vi "RFID MFRC522 Example.vi"   [LabVIEW 2014]
doc: "This example shows how read/write data to RFID tag (MFRC522)"
uses:
  QwaveSys_Interface/QwaveSys_Interface.lvlib
  PWS_ESP8266/PWS_ESP8266.lvlib
panel:
  # "Overview: Demonstrates how to read communicate with contactless reader/writer RFID NXP MFRC522.\nRequirements: LabVIEW Full Development System,Arduino Compatible Compiler for LabVIEW,Programmable Wireless Stamp (PWS) Library.\nInstructions:\n1. Plug-in RFID MFRC522 module  to SPI port refer diagram below.\n2.  If this example has been loaded from the Arduino Compatible Compiler for LabVIEW, simply select Compile and Download.  Otherwise, open Tools>Arduino Compatible Compiler for LabVIEW in LabVIEW, then select File>Load VI, and select this VI and then Compile and Download.\n3. Open \"Serial Monitor\" by select \"Tools>Serial Monitor\" and select baud rate to 9600.\n4. Observe the logged data being print out on serial port monitor. \n\n#NOTE: \nThe MFRC522 is an integrated reader/writer integrated circuit for contactless communication at 13.56 MHz, by NXP technologies. refer : \"http://www.nxp.com/products/identification-and-security/nfc-and-reader-ics/nfc-frontend-solutions/standard-3v-mifare-reader-solution:MFRC522\""
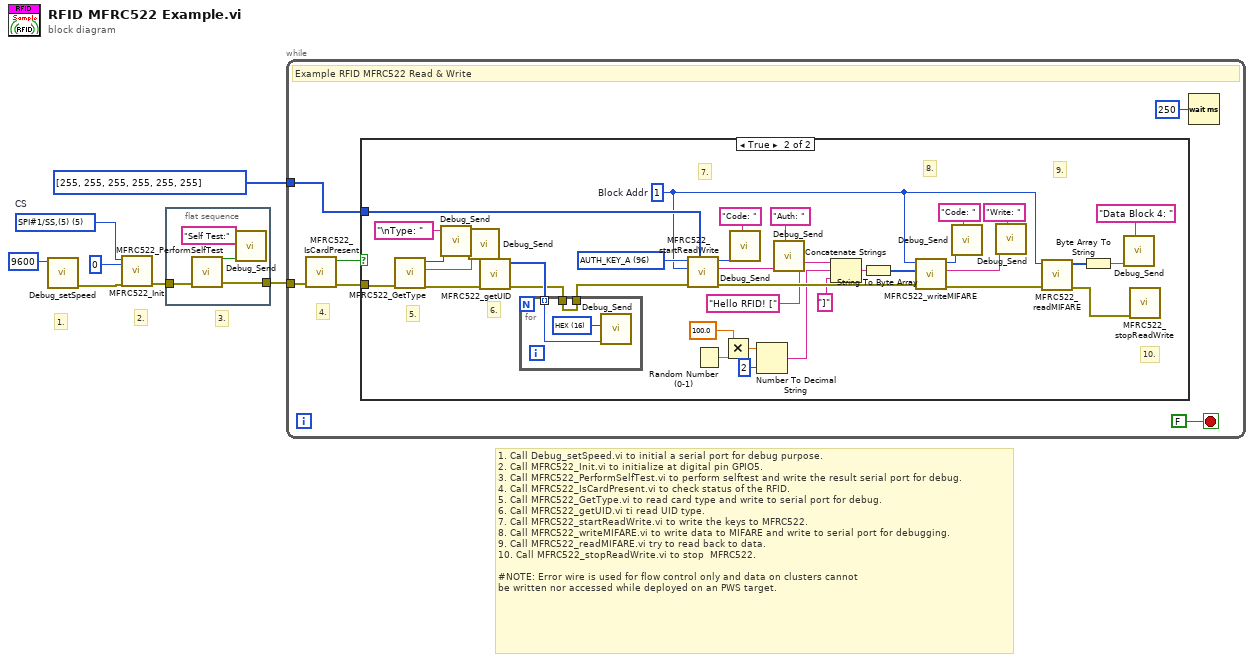
[diagram p0: block diagram]
diagram:
  w1 = u8 5 items=["SPI#1/SS,(5)"=5, "SPI#2/MOSI,(13)"=13, "SPI#3/MISO,(12)"=12, "SPI#4/SCLK,(14)"=14, "UART#1/CS,(15)"=15, "UART#2/TXD,(1)"=1, "UART#3/RXD,(3)"=3, "UART#4/LED,(16)"=16, "FPROM_Btn,(0)"=0, "SDCard_CS,(4)"=4, "I2C-SDA/TXD1,(2)"=2, "ADC0,(17)"=17]  # CS
  # "1. Call Debug_setSpeed.vi to initial a serial port for debug purpose.\n2. Call MFRC522_Init.vi to initialize at digital pin GPIO5.\n3. Call MFRC522_PerformSelfTest.vi to perform selftest and write the result serial port for debug.\n4. Call MFRC522_IsCardPresent.vi to check status of the RFID.\n5. Call MFRC522_GetType.vi to read card type and write to serial port for debug.\n6. Call MFRC522_getUID.vi ti read UID type.\n7. Call MFRC522_startReadWrite.vi to write the keys to MFRC522.\n8. Call MFRC522_writeMIFARE.vi to write data to MIFARE and write to serial port for debugging.\n9. Call MFRC522_readMIFARE.vi try to read back to data.\n10. Call MFRC522_stopReadWrite.vi to stop  MFRC522.\n\n#NOTE: Error wire is used for flow control only and data on clusters cannot\nbe written nor accessed while deployed on an PWS target."
  # "3."
  # "2."
  # "1."
  n1 = call "Debug_setSpeed.vi"("Speed"=u32 9600) -> ("error out"=w6:errorcluster)  [unwired: 10 in]
  n2 = call "MFRC522_Init.vi"("error in (no error)"=w6, "Reset"=u8 0, "Chip Select"=w1) -> ("error out"=w3:errorcluster)  [unwired: 8 in]
  n3 = flat-sequence {
    tunnel: w3 -> [w10]
    tunnel: [w9] -> w2
    frame #0 {
      n4 = call "MFRC522_PerformSelfTest.vi"("error in (no error)"=w10) -> ("error out"=w9:errorcluster, "status"=w8:bool)  [unwired: 9 in]
      n5 = call "Debug_Send.vi"("Name"="Self Test:", "DATA"=w8) -> ()  [unwired: 10 in]
    }
  }
  n6 = while {
    tunnel: w2 -> [w17]
    tunnel: u8[] [255, 255, 255, 255, 255, 255] ("Key (6 bytes)") -> [w12]
    stop <- FALSE stop-if-true
    # "4."
    # "Example RFID MFRC522 Read & Write"
    n7 = call "MFRC522_IsCardPresent.vi"("error in (no error)"=w17) -> ("error out"=w16:errorcluster, "status"=w13:bool)  [unwired: 9 in]
    n8 = case shown="True" w13 {
      tunnel: w16 -> [_ w36]
      tunnel: w12 -> [_ w49]
      frame False {
      }
      frame True {
        w18 = u8 1  # Block Addr
        w51 = u16 96 items=["AUTH_KEY_A"=96, "AUTH_KEY_B"=97] ("Key")
        # "10."
        # "9."
        # "8."
        # "7."
        # "6."
        # "5."
        n9 = call "MFRC522_GetType.vi"("error in (no error)"=w36) -> ("error out"=w35:errorcluster, "Type Name"=w32:string, "Type"=w33:u8)  [unwired: 8 in]
        n10 = call "Debug_Send.vi"("Name"="\nType: ", "DATA"=w33) -> ()  [unwired: 10 in]
        n11 = call "Debug_Send.vi"("DATA"=w32) -> ()  [unwired: 11 in]
        n12 = call "MFRC522_getUID.vi"("error in (no error)"=w35) -> ("error out"=w20:errorcluster, "UID"=w34:u8[])  [unwired: 9 in]
        n13 = for {
          tunnel: w34 -> [w54] mode=indexing
          tunnel: w20 -> [w52]
          tunnel: [w52] -> w19
          w53 = u16 16 items=["DEC"=10, "HEX"=16, "OCT"=8, "BIN"=2] ("Option")
          n14 = call "Debug_Send.vi"("DATA"=w54, "Option"=w53) -> ()  [unwired: 10 in]
        }
        n15 = call "MFRC522_startReadWrite.vi"("Key (6 bytes)"=w49, "error in (no error)"=w19, "Block Address"=w18, "Key"=w51) -> ("error out"=w46:errorcluster, "Status Name"=w30:string, "Status Code"=w29:u8)  [unwired: 5 in]
        n16 = Random Number (0-1)() -> (number: 0 to 1=w44:dbl)
        n17 = Multiply(x=100.0, y=w44) -> (x*y=w42:dbl)
        n18 = call "Debug_Send.vi"("Name"="Code: ", "DATA"=w29) -> ()  [unwired: 10 in]
        n19 = Number To Decimal String(number=w42, width (-)=i16 2) -> (decimal integer string=w40:string)
        n20 = call "Debug_Send.vi"("Name"="Auth: ", "DATA"=w30) -> ()  [unwired: 10 in]
        n21 = Concatenate Strings("Hello RFID! [", w40, "]" ("string")) -> (w38:string)
        n22 = String To Byte Array(string=w38) -> (unsigned byte array=w45:u8[])
        n23 = call "MFRC522_writeMIFARE.vi"("error in (no error)"=w46, "Data (max 16 bytes)"=w45, "Block Address"=w18) -> ("error out"=w47:errorcluster, "Status Name"=w23:string, "Status Code"=w26:u8)  [unwired: 6 in]
        n24 = call "Debug_Send.vi"("Name"="Code: ", "DATA"=w26) -> ()  [unwired: 10 in]
        n25 = call "Debug_Send.vi"("Name"="Write: ", "DATA"=w23) -> ()  [unwired: 10 in]
        n26 = call "MFRC522_readMIFARE.vi"("error in (no error)"=w47, "Block Address"=w18) -> ("error out"=w50:errorcluster, "Data"=w48:u8[])  [unwired: 8 in]
        n27 = Byte Array To String(unsigned byte array=w48) -> (string=w22:string)
        n28 = call "Debug_Send.vi"("Name"="Data Block 4: ", "DATA"=w22) -> ()  [unwired: 10 in]
        n29 = call "MFRC522_stopReadWrite.vi"("error in (no error)"=w50) -> ()  [unwired: 10 in, 1 out]
      }
    }
    n30 = Wait (ms)(milliseconds to wait=u32 250) -> ()  [unwired: 1 out]
  }
